vi "DispenseOff.vi"(8 "error in (no error)":errorcluster, 11 "I-O in":refnum<class "Copy of I-O.lvclass">) -> (0 "error out":errorcluster, 3 "I-O out":refnum<class "Copy of I-O.lvclass">)   [LabVIEW 2016]
uses:
  Copy of I-O.lvclass
panel:
  # "Set Dispense Off"
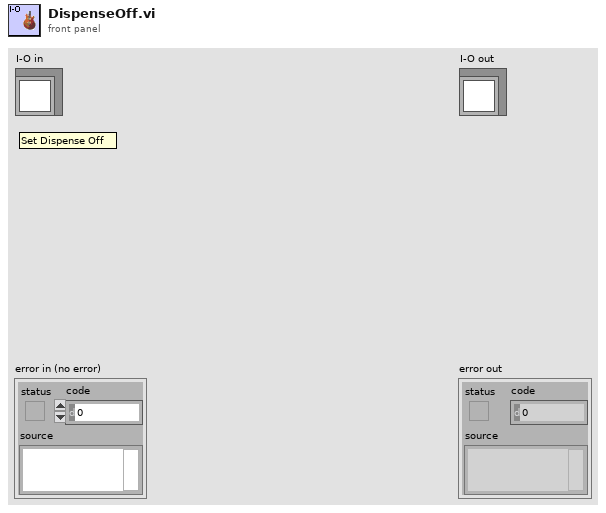
[diagram p1: front panel]
types:
  T1 = typedef "Copy of I-O.lvclass/Pin Map.ctl" = cluster{"Region Valves":i32[], "Extra Valves":dbl[][], "Tool Primary Valve":i32, "Tool Secondary Valve":i32, "Region Sensors":i32[], "Extra Sensors":dbl[][], "Tool Primary Sensor":dbl, "Tool Secondary Sensor":dbl, "Compression Sensor":dbl, "5V":i32, "NTU_Glue":dbl}
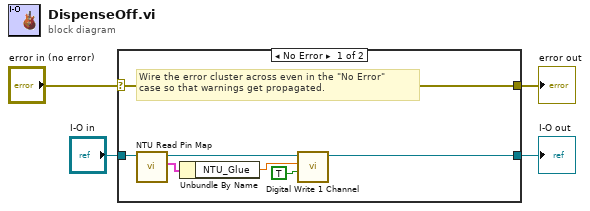
[diagram p0: block diagram]
diagram:
  n1 = case shown="No Error" "error in (no error)" {
    selector: "error in (no error)" -> [w11 w13]
    tunnel: [w11 w13] -> w3
    tunnel: [w9 w12] -> w1
    tunnel: "I-O in" -> [w8 w12]
    frame No Error {
      # "Wire the error cluster across even in the \"No Error\"\ncase so that warnings get propagated."
      n2 = call-dynamic "NTU Read Pin Map.vi"("I-O in"=w8) -> ("Pin Map"=w5:T1, "I-O out"=w7:refnum<class "Copy of I-O.lvclass">)  [unwired: 8 in, 1 out]
      n3 = Unbundle By Name(w5) -> ("NTU_Glue"=w6:dbl)
      n4 = call-dynamic "Digital Write 1 Channel.vi"("Value"=TRUE, "Channel"=w6, "I-O.lvclass"=w7) -> ("I-O.lvclass 2"=w9:refnum<class "Copy of I-O.lvclass">)  [unwired: 7 in, 1 out]
    }
    frame Error {
    }
  }
  "error out" <- w3
  "I-O out" <- w1
